vi "test.vi"() -> ()   [LabVIEW 2021]
uses:
  <vilib>/Instr/_visa.llb/VISA Configure Serial Port (Instr).vi
panel:
  out "Prueba 5V":bool
  out "5V":string
  out "Tensión 1":dbl format="%_3g"
  out "I/O":string
  out "appended array":i32[](array[numeric])
  out "Prueba I/O":bool
  out "Prueba 1V8":bool
  out "1V8":string
  out "Tensión 3":dbl format="%_3g"
  out "Prueba 3V3":bool
  out "3V3":string
  out "Tensión 2":dbl format="%_3g"
  in  "stop":bool
  out "Slide":u8(slide) scale=0.0..100.0
  # "Prueba de validaciÃ³n de placa basada en CPLDón de PCB basada en CPLD"
  # "Error en pin(es):"
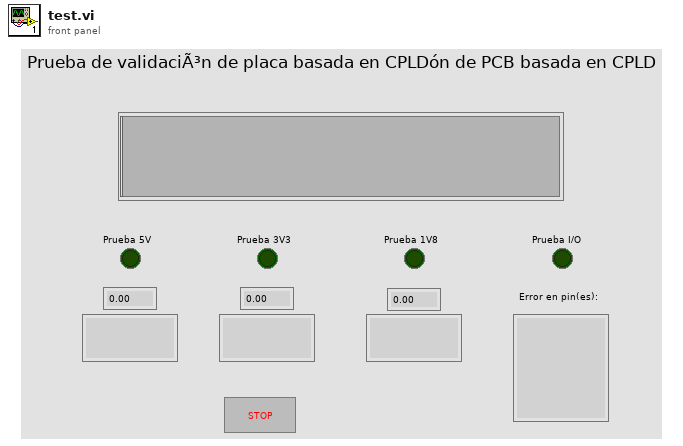
[diagram p1: front panel]
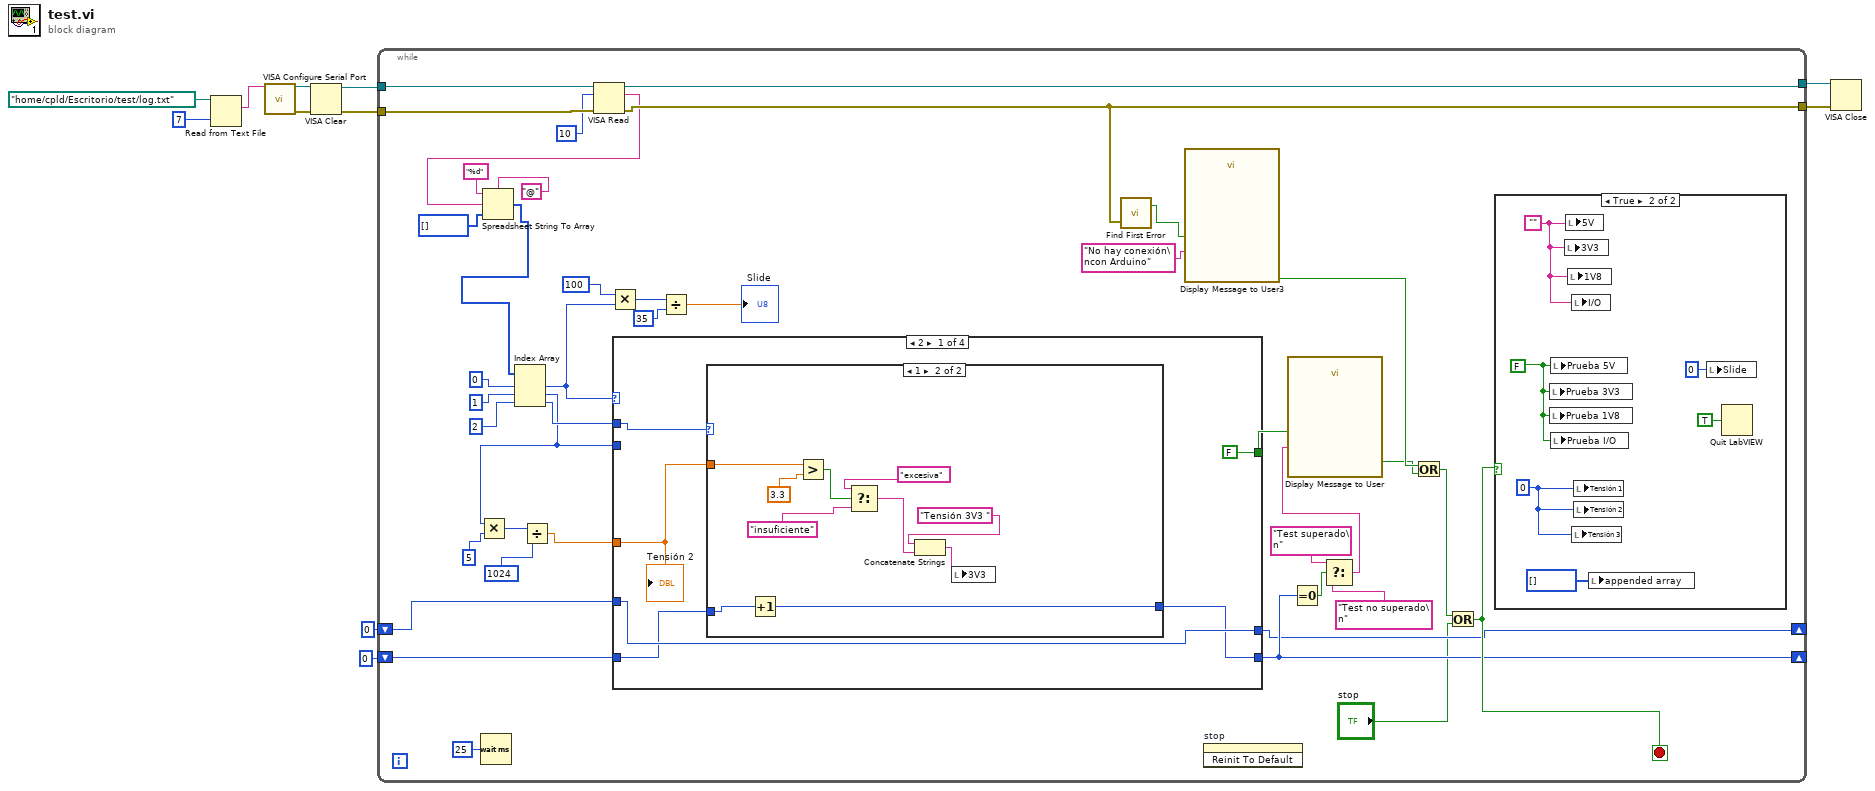
[diagram p0: block diagram]
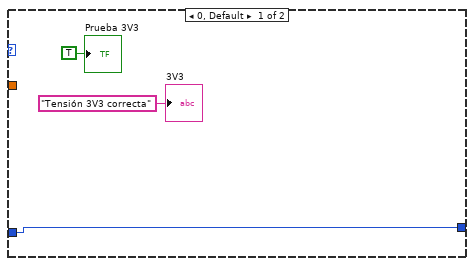
[diagram p2: hidden frame]
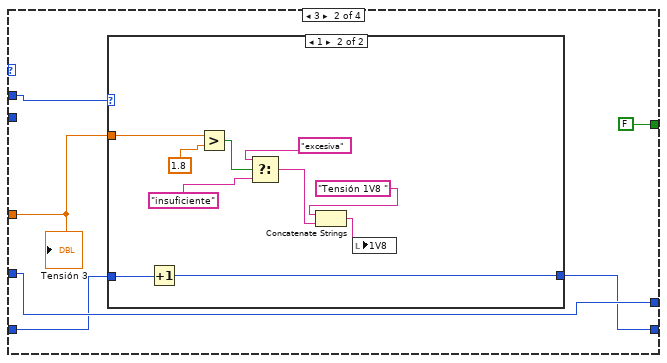
[diagram p3: hidden frame]
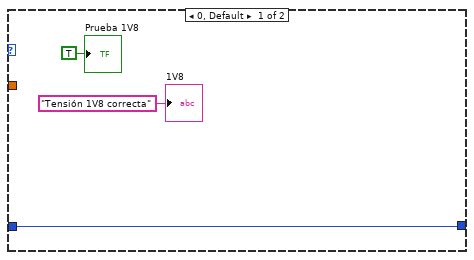
[diagram p4: hidden frame]
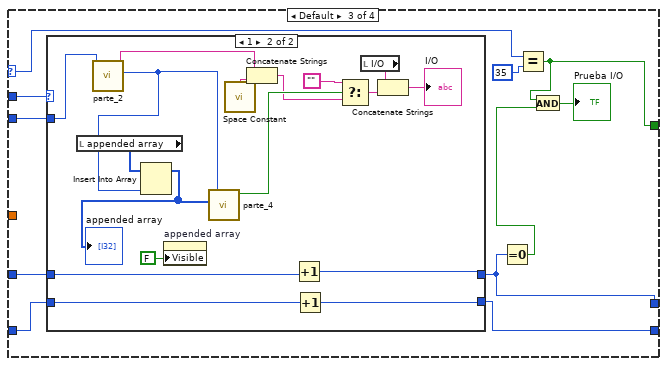
[diagram p5: hidden frame]
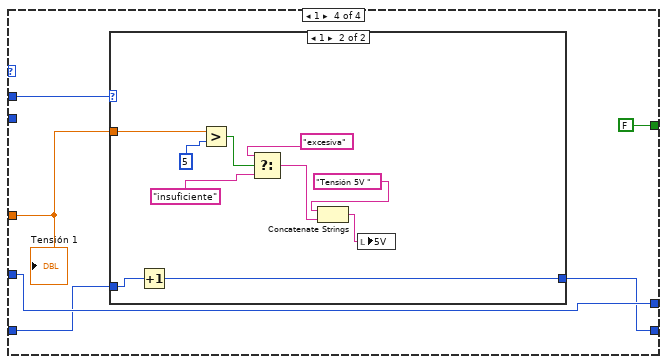
[diagram p7: hidden frame]
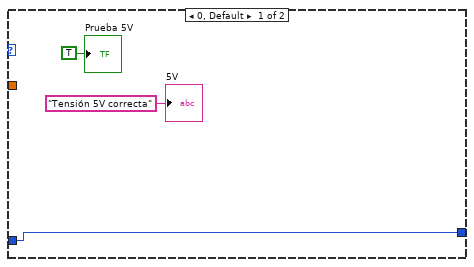
[diagram p8: hidden frame]
diagram:
  n1 = Read from Text File(file (use dialog)=path "/home/cpld/Escritorio/test/log.txt", count=7) -> (text=w2:string)  [unwired: 2 in, 3 out]
  n2 = call-poly "VISA Configure Serial Port"("VISA resource name"=w2) -> ("VISA resource name out"=w5:refnum<visa-resource-name>, "error out"=w6:errorcluster)  [unwired: 13 in]
  n3 = VISA Clear(VISA resource name=w5, error in (no error)=w6) -> (VISA resource name out=w4:refnum<visa-resource-name>, error out=w3:errorcluster)
  n4 = while {
    tunnel: [w17] -> w11
    shift-right: [w24] -> _
    shift-left: u32 0 ("milliseconds to wait") -> [w32]
    tunnel: w4 -> [w19]
    tunnel: w3 -> [w20]
    tunnel: [w16] -> w10
    shift-right: [w23] -> _
    shift-left: u32 0 ("milliseconds to wait") -> [w31]
    stop <- w41 stop-if-true
    n5 = Wait (ms)(milliseconds to wait=u32 25) -> ()  [unwired: 1 out]
    n6 = VISA Read(VISA resource name=w19, byte count=u32 10, error in (no error)=w20) -> (VISA resource name out=w17:refnum<visa-resource-name>, read buffer=w14:string, error out=w16:errorcluster)  [unwired: 1 out]
    n7 = Spreadsheet String To Array(delimiter (Tab)="@" ("search string/char (-)"), format string="%d", spreadsheet string=w14, array type (2D Dbl)=i32[] []) -> (array=w13:i32[])
    n8 = Index Array(array=w13, index #1=0 ("index"), index #2=1 ("index"), index #3=2 ("index")) -> (element #1=w30:i32, element #2=w22:i32, element #3=w29:i32)
    n9 = Multiply(x=w22, y=u8 5 ("x")) -> (x*y=w28:i32)
    n10 = Divide(x=w28, y=u16 1024) -> (x/y=w25:dbl)
    n11 = Multiply(x=u8 100, y=w30) -> (x*y=w52:i32)
    n12 = case shown="2" w30 {
      selector: w30 -> [_ _ w96 _]
      tunnel: w29 -> [w57 w76 w101 w126]
      tunnel: w25 -> [w58 w77 _ w125]
      tunnel: w31 -> [w56 w75 w100 w124]
      tunnel: [w56 w75 w91 w124] -> w23
      tunnel: w22 -> [_ _ w97 _]
      tunnel: w32 -> [w55 w74 w99 w123]
      tunnel: [w54 w73 w98 w122] -> w24
      tunnel: [FALSE FALSE w94 FALSE] -> w38
      frame 2 {
        n13 = case shown="1" w57 {
          tunnel: w58 -> [_ w65]
          tunnel: w55 -> [w60 w64]
          tunnel: [w60 w63] -> w54
          frame 0, Default {
            "Prueba 3V3" <- TRUE
            "3V3" <- "Tensión 3V3 correcta" ("3V3")
          }
          frame 1 {
            n14 = Increment(x=w64) -> (x+1=w63:u32)
            n15 = Greater?(x=w65, y=3.3 ("x")) -> (0:w70:bool)
            n16 = Select(t="excesiva" ("read buffer 2"), s=w70, f="insuficiente") -> (s? t:f=w66:string)
            n17 = Concatenate Strings("Tensión 3V3 " ("string"), w66) -> (w67:string)
            n18 = local write "3V3"(w67) -> ()
          }
        }
        "Tensión 2" <- w58
      }
      frame 3 {
        n19 = case shown="1" w76 {
          tunnel: w77 -> [_ w84]
          tunnel: w74 -> [w79 w83]
          tunnel: [w79 w82] -> w73
          frame 0, Default {
            "Prueba 1V8" <- TRUE
            "1V8" <- "Tensión 1V8 correcta" ("1V8")
          }
          frame 1 {
            n20 = Increment(x=w83) -> (x+1=w82:u32)
            n21 = Greater?(x=w84, y=1.8 ("x")) -> (0:w89:bool)
            n22 = Select(t="excesiva" ("read buffer 2"), s=w89, f="insuficiente") -> (s? t:f=w85:string)
            n23 = Concatenate Strings("Tensión 1V8 " ("string"), w85) -> (w86:string)
            n24 = local write "1V8"(w86) -> ()
          }
        }
        "Tensión 3" <- w77
      }
      frame Default {
        n25 = case shown="1" w101 {
          tunnel: [w103 w119] -> w91
          tunnel: w100 -> [w103 w120]
          tunnel: w97 -> [_ w106]
          tunnel: w99 -> [w102 w105]
          tunnel: [w102 w104] -> w98
          frame 0, Default {
          }
          frame 1 {
            n26 = local read "appended array"() -> (w116:i32[])
            n27 = call "parte_2.vi"("info"=w106) -> ("pin_int"=w111:i32, "pin_string"=w113:string)  [unwired: 9 in]
            n28 = Insert Into Array(array=w116, new element=w111) -> (w109:i32[])  [unwired: 1 in]
            "appended array" <- w109
            n29 = property on="appended array" class="Arr (strict)"("Visible"=FALSE) -> ()  [unwired: 2 in, 2 out]
            n30 = call "parte_4.vi"("array"=w109, "error_pin"=w111) -> ("Boolean"=w110:bool)  [unwired: 9 in]
            n31 = call <vilib>:"Space Constant.vi"() -> ("String"=w114:string)
            n32 = Concatenate Strings(w113, w114) -> (w107:string)
            n33 = Increment(x=w120) -> (x+1=w119:u32)
            n34 = Increment(x=w105) -> (x+1=w104:u32)
            n35 = Select(t="", s=w110, f=w107) -> (s? t:f=w112:string)
            n36 = local read "I/O"() -> (w118:string)
            n37 = Concatenate Strings(w118, w112) -> (→"I/O":string)
          }
        }
        n38 = Equal To 0?(x=w91) -> (x = 0?=w95:bool)
        n39 = Equal?(x=w96, y=35) -> (x = y?=w94:bool)
        n40 = And(x=w94, y=w95) -> (x .and. y?=→"Prueba I/O":bool)
      }
      frame 1 {
        n41 = case shown="1" w126 {
          tunnel: w125 -> [_ w133]
          tunnel: w123 -> [w128 w132]
          tunnel: [w128 w131] -> w122
          frame 0, Default {
            "Prueba 5V" <- TRUE
            "5V" <- "Tensión 5V correcta" ("5V")
          }
          frame 1 {
            n42 = Increment(x=w132) -> (x+1=w131:u32)
            n43 = Greater?(x=w133, y=u8 5 ("x")) -> (0:w138:bool)
            n44 = Select(t="excesiva" ("read buffer 2"), s=w138, f="insuficiente") -> (s? t:f=w134:string)
            n45 = Concatenate Strings("Tensión 5V " ("string"), w134) -> (w135:string)
            n46 = local write "5V"(w135) -> ()
          }
        }
        "Tensión 1" <- w125
      }
    }
    n47 = Divide(x=w52, y=35) -> (x/y=→"Slide":dbl)
    n48 = call <vilib>:"Find First Error.vi"("error in (no error)"=w16) -> ("error?"=w42:bool)  [unwired: 3 in, 1 out]
    n49 = call "Display Message to User3"("Enable"=w42, "Message"="No hay conexión\ncon Arduino") -> ("OK"=w40:bool)  [unwired: 8 in, 1 out]
    n50 = invoke on="stop" class="Bool (strict)" method="Reinit To Default"() -> ()  [unwired: 3 in, 3 out]
    n51 = Equal To 0?(x=w24) -> (x = 0?=w35:bool)
    n52 = Select(t="Test superado\n" ("Message"), s=w35, f="Test no superado\n" ("Message")) -> (s? t:f=w36:string)
    n53 = call "Display Message to User"("Enable"=w38, "Message"=w36) -> ("OK"=w34:bool)  [unwired: 8 in, 1 out]
    n54 = Or(x=w40, y=w34) -> (x .or. y?=w39:bool)
    n55 = Or(x=w39, y="stop") -> (x .or. y?=w41:bool)
    n56 = case shown="True" w41 {
      frame False {
      }
      frame True {
        w142 = ""
        w140 = 0
        w143 = FALSE
        n57 = local write "Prueba 3V3"(w143) -> ()
        n58 = local write "Prueba 1V8"(w143) -> ()
        n59 = local write "Prueba 5V"(w143) -> ()
        n60 = local write "Prueba I/O"(w143) -> ()
        n61 = local write "3V3"(w142) -> ()
        n62 = local write "5V"(w142) -> ()
        n63 = local write "1V8"(w142) -> ()
        n64 = local write "I/O"(w142) -> ()
        n65 = local write "Tensión 3"(w140) -> ()
        n66 = local write "Tensión 1"(w140) -> ()
        n67 = local write "Tensión 2"(w140) -> ()
        n68 = local write "appended array"(i32[] []) -> ()
        n69 = local write "Slide"(u8 0 ("Slide")) -> ()
        n70 = Quit LabVIEW(quit? (T)=TRUE) -> ()
      }
    }
  }
  n71 = VISA Close(VISA resource name=w11, error in (no error)=w10) -> ()  [unwired: 1 out]
